vi "Data_reduction.vi"(6 "Offset":i16, 7 "Reduce data? in":bool, 8 "Master?":bool, 9 "Length":u16, 10 "Cut off":i16, 11 "Data in":u8[](array[numeric])) -> (0 "Reduce data? out":bool, 1 "Length":u16, 2 "Data out":u8[](array[numeric]))   [LabVIEW 2013]
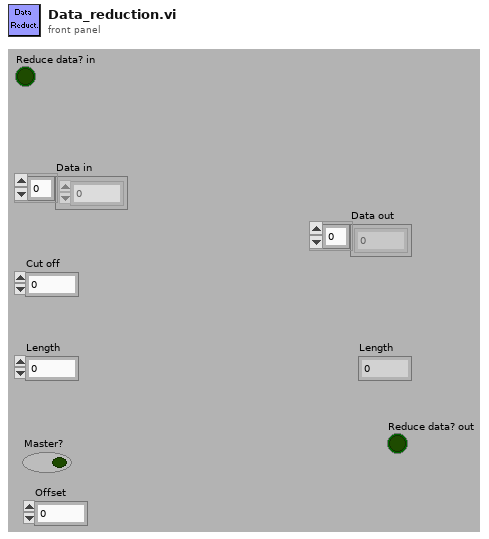
[diagram p1: front panel]
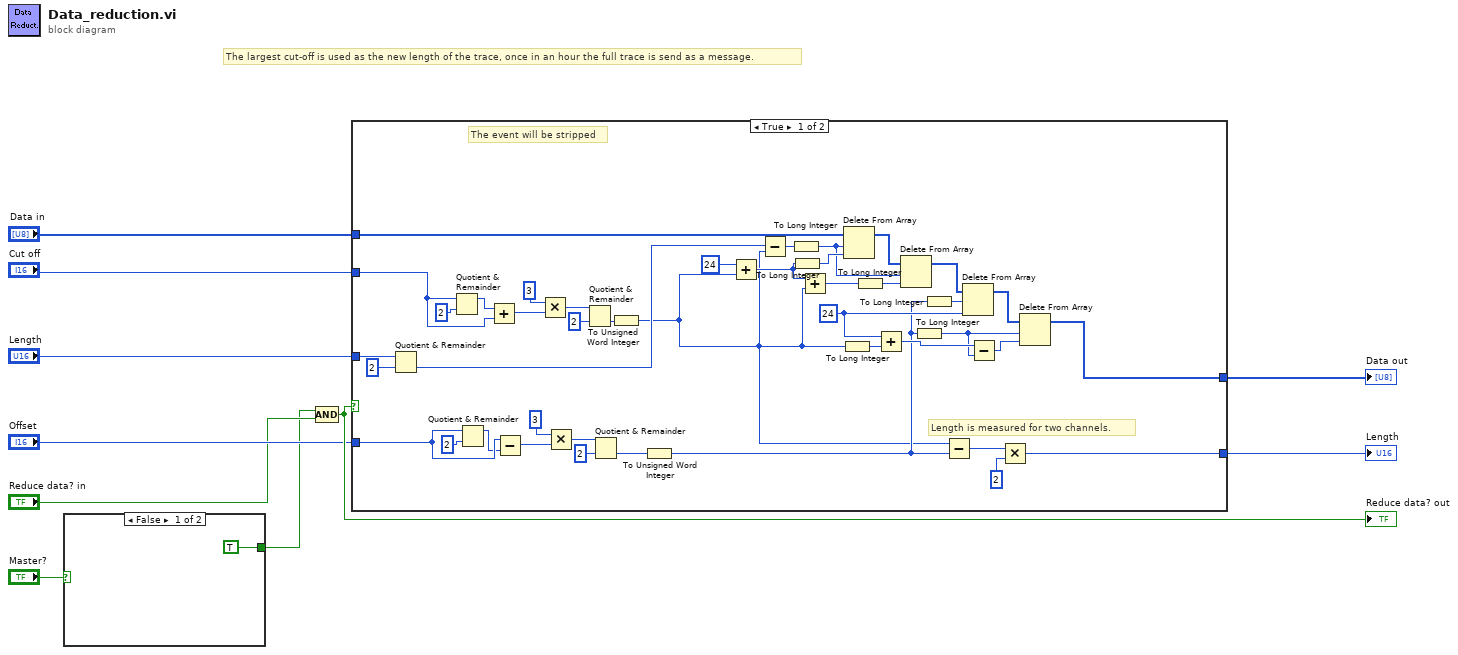
[diagram p0: block diagram]
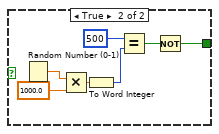
[diagram p2: hidden frame]
diagram:
  # "The largest cut-off is used as the new length of the trace, once in an hour the full trace is send as a message."
  n1 = case shown="False" "Master?" {
    tunnel: [TRUE w12] -> w2
    frame False {
    }
    frame True {
      n2 = Random Number (0-1)() -> (number: 0 to 1=w18:dbl)
      n3 = Multiply(x=w18, y=1000.0) -> (x*y=w16:dbl)
      n4 = To Word Integer(number=w16) -> (16bit integer=w15:i16)
      n5 = Equal?(x=i16 500, y=w15) -> (x = y?=w13:bool)
      n6 = Not(x=w13) -> (.not. x?=w12:bool)
    }
  }
  n7 = Compound Arithmetic op=AND(w2, "Reduce data? in") -> (w5:bool)
  "Reduce data? out" <- w5
  n8 = case shown="True" w5 {
    tunnel: "Cut off" -> [w37 _]
    tunnel: [w46 w62] -> w9
    tunnel: "Length" -> [w45 w62]
    tunnel: [w49 w61] -> w7
    tunnel: "Data in" -> [w43 w61]
    tunnel: "Offset" -> [w25 _]
    frame True {
      w34 = 24 ("x")
      # "Length is measured for two channels."
      # "The event will be stripped"
      n9 = Quotient & Remainder(x=w45, y=u16 2) -> (floor(x/y)=w38:u16)  [unwired: 1 out]
      n10 = Quotient & Remainder(x=w37, y=i16 2 ("x")) -> (x-y*floor(x/y)=w36:i16)  [unwired: 1 out]
      n11 = Quotient & Remainder(x=w25, y=i16 2 ("x")) -> (x-y*floor(x/y)=w24:i16)  [unwired: 1 out]
      n12 = Add(x=w36, y=w37) -> (x+y=w35:i16)
      n13 = Subtract(x=w25, y=w24) -> (x-y=w28:i16)
      n14 = Multiply(x=i16 3, y=w35) -> (x*y=w40:i16)
      n15 = Multiply(x=i16 3, y=w28) -> (x*y=w30:i16)
      n16 = Quotient & Remainder(x=w40, y=i16 2 ("x")) -> (floor(x/y)=w27:i16)  [unwired: 1 out]
      n17 = Quotient & Remainder(x=w30, y=i16 2 ("x")) -> (floor(x/y)=w26:i16)  [unwired: 1 out]
      n18 = To Unsigned Word Integer(number=w27) -> (unsigned 16bit integer=w19:u16)
      n19 = To Unsigned Word Integer(number=w26) -> (unsigned 16bit integer=w21:u16)
      n20 = Add(x=u16 24, y=w19) -> (x+y=w55:u16)
      n21 = Subtract(x=w38, y=w19) -> (x-y=w59:u16)
      n22 = To Long Integer(number=w59) -> (32bit integer=w56:i32)
      n23 = To Long Integer(number=w55) -> (32bit integer=w58:i32)
      n24 = Add(x=w55, y=w19) -> (x+y=w54:u16)
      n25 = To Long Integer(number=w19) -> (32bit integer=w50:i32)
      n26 = Delete From Array(array=w43, length=w56, index=w58) -> (array with subset deleted=w57:u8[])  [unwired: 1 out]
      n27 = To Long Integer(number=w54) -> (32bit integer=w53:i32)
      n28 = Add(x=w34, y=w50) -> (x+y=w23:i32)
      n29 = Delete From Array(array=w57, length=w56, index=w53) -> (array with subset deleted=w51:u8[])  [unwired: 1 out]
      n30 = To Long Integer(number=w21) -> (32bit integer=w20:i32)
      n31 = To Long Integer(number=w21) -> (32bit integer=w33:i32)
      n32 = Subtract(x=w19, y=w21) -> (x-y=w48:u16)
      n33 = Delete From Array(array=w51, length=w33, index=w34) -> (array with subset deleted=w52:u8[])  [unwired: 1 out]
      n34 = Subtract(x=w23, y=w20) -> (x-y=w22:i32)
      n35 = Multiply(x=w48, y=u16 2) -> (x*y=w46:u16)
      n36 = Delete From Array(array=w52, length=w20, index=w22) -> (array with subset deleted=w49:u8[])  [unwired: 1 out]
    }
    frame False {
      # "This is the first event this hour, or there is more than one peak in one of the channels, it will not be stripped"
    }
  }
  "Data out" <- w7
  "Length" <- w9
